vi "T_At_Wire_I32.vi"(8 "InitClock(ms)":u32, 11 "I32":i32) -> (0 "Clock(ms)":u32, 3 "I32 Out":i32, 4 "Delta(ms)":u32)   [LabVIEW 2019]
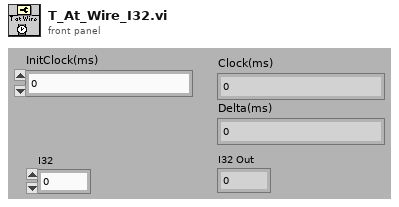
[diagram p1: front panel]
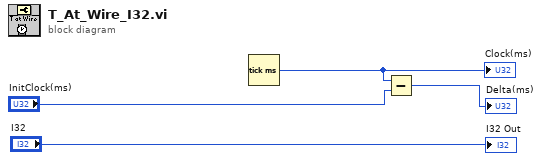
[diagram p0: block diagram]
diagram:
  n1 = Tick Count (ms)() -> (millisecond timer value=w2:u32)
  "Clock(ms)" <- w2
  n2 = Subtract(x=w2, y="InitClock(ms)") -> (x-y=→"Delta(ms)":u32)
  "I32 Out" <- "I32"
